vi "LINX - PWM 1 Channel.vi"() -> ()   [LabVIEW 2014, in "LMH-LINX.lvlib"]
doc: "This example demonstrates how to generate a PWM signal on a single channel using a LINX device."
uses:
  vi.lib/MakerHub/LINX/LMH-LINX.lvlib
  vi.lib/MakerHub/LINX/Public/Peripherals/PWM/PWM Set Duty Cycle 1 Chan.vi
  vi.lib/MakerHub/LINX/Public/Utilities/Open Serial.vi
  vi.lib/MakerHub/LINX/Public/Peripherals/PWM/PWM Set Duty Cycle N Chans.vi
panel:
  in  "Duty Cycle (0-1)":dbl
  in  "PWM Channel":u8=3
  in  "Stop Button":bool
  in  "Serial Port":refnum<visa-resource-name>
  # "LINX Device Settings"
  # "PWM 1 Channel Example\n\nThis example demonstrates how to set the dutry cycle of one PWM channel.\nA duty cycle of 0 coresponds to 0% on and a duty cycle of 1 coresponds to 100% on.\n\nInstructions\n1. Select the COM Port associated with the LINX Device.\n2. Select the PWM Channels to write to.\n3. Click the Run Arrow."
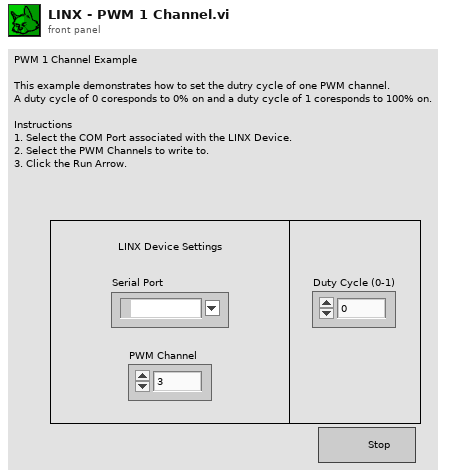
[diagram p1: front panel]
types:
  T1 = typedef "LMH-LINX.lvlib/LINX Ref.ctl" = cluster{"IO":T2, "Interface":T3, "LINX Device Config":T4}
  T2 = typedef "LMH-LINX.lvlib/Platform.ctl" = enum16{"Remote", "Local"}
  T3 = typedef "LMH-LINX.lvlib/Interface.ctl" = enum16{"Serial", "TCP"}
  T4 = typedef "LMH-LINX.lvlib/Device.lvlib/LINX Device Config.ctl" = cluster{"Interface":T3, "COM Port":refnum<visa-resource-name>, "TCP Configuration":T5, "Device Family":u8, "Device ID":u8, "Device Name":string, "TCP Ref":refnum<k5>, "Channels":T6}
  T5 = typedef "LMH-LINX.lvlib/Device.lvlib/TCP Config.ctl" = cluster{"IP Address":string, "Port":u16}
  T6 = typedef "LMH-LINX.lvlib/Channels.ctl" = cluster{"DI":u8[], "DO":u8[], "AI":u8[], "AO":u8[], "PWM":u8[], "QE":u8[], "UART":u8[], "I2C 2":u8[], "SPI":u8[], "CAN":u8[], "Servo":u8[], "AI Ref (V)":dbl, "AI Resolution (Bits)":u8, "AO Ref (V)":dbl, "AO Resolution (Bits)":u8}
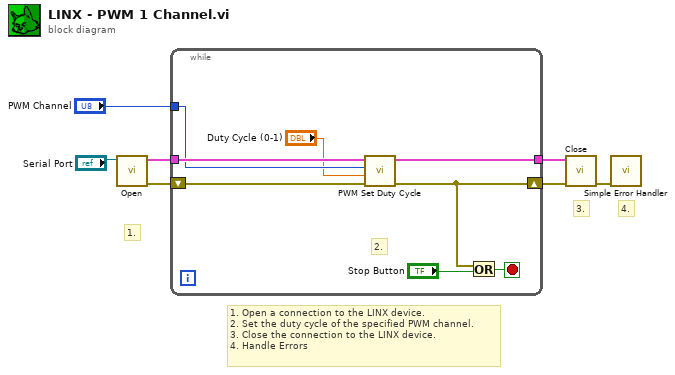
[diagram p0: block diagram]
diagram:
  # "1. Open a connection to the LINX device.\n2. Set the duty cycle of the specified PWM channel.\n3. Close the connection to the LINX device.\n4. Handle Errors"
  # "4."
  # "3."
  # "1."
  n1 = call-poly "Open.vi"("Serial Port"="Serial Port") -> ("Error Out"=w6:errorcluster, "LINX Resource"=w7:T1)  [unwired: 8 in, 1 out]
  n2 = while {
    tunnel: w7 -> [w11]
    tunnel: [w10] -> w5
    shift-right: [w12] -> w4
    shift-left: w6 -> [w13]
    tunnel: "PWM Channel" -> [w9]
    stop <- w15 stop-if-true
    # "2."
    n3 = call-poly "PWM Set Duty Cycle.vi"("Error In"=w13, "Duty Cycle (0-1)"="Duty Cycle (0-1)", "PWM Channel"=w9, "LINX Resource"=w11) -> ("Error Out"=w12:errorcluster, "LINX Resource"=w10:T1)  [unwired: 6 in]
    n4 = Or(x=w12, y="Stop Button") -> (x .or. y?=w15:bool)
  }
  n5 = call "Close.vi"("Error In"=w4, "LINX Resource"=w5) -> ("Error Out"=w2:errorcluster)  [unwired: 9 in]
  n6 = call <vilib>:"Simple Error Handler.vi"("error in (no error)"=w2) -> ()  [unwired: 4 in, 5 out]
